vi "Query Sequencer Reliability.vi"(8 "error in (no error)":errorcluster, 10 "Instance (1)":i32=1, 11 "VISA resource name":refnum<visa-resource-name>) -> (0 "error out":errorcluster, 1 "Reliability Message":string, 2 "Reliability":i32, 3 "VISA resource name out":refnum<visa-resource-name>, 4 "Additional Info":string)   [LabVIEW 2015, in "Rohde&Schwarz CMXP GPRF.lvlib"]
doc: "Reports if and why there are problems generating the configured signal.\n\nAttribute:\nRSCMXPGPRF_ATTR_SEQUENCER_RELIABILITY\n\nRemote-control command:\nSOURce:GPRF:GEN<i>:SEQuencer:RELiability:ALL?"
uses:
  <instrlib>/Rohde&Schwarz CMXP GPRF/Rohde&Schwarz CMXP GPRF.lvlib
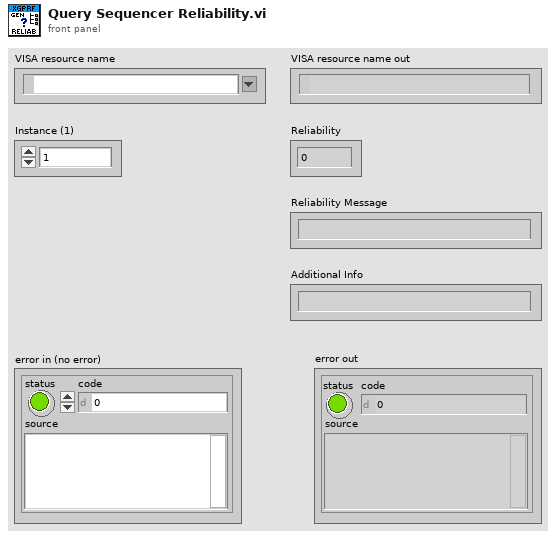
[diagram p1: front panel]
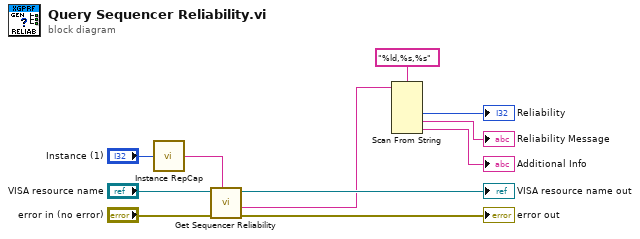
[diagram p0: block diagram]
diagram:
  n1 = call <instrlib>:"Instance RepCap.vi"("instance  in"="Instance (1)") -> ("instance out"=w4:string)
  n2 = call "Get Sequencer Reliability"("Repeated Capabilities"=w4, "error in (no error)"="error in (no error)", "instrument handle"="VISA resource name") -> ("error out"=→"error out":errorcluster, "Sequencer Reliability"=w3:string, "instrument handle out"=→"VISA resource name out":refnum<visa-resource-name>)  [unwired: 6 in]
  n3 = Scan From String(format string="%ld,%s,%s", input string=w3) -> (output 1=→"Reliability":i32, output 2=→"Reliability Message":string, output 3=→"Additional Info":string)  [unwired: 5 in, 3 out]
